vi "SaveDataToDiskAsGlimpse.vi"(0 "Read or Write Path":path, 1 "Array (U8)":u8[][](array[numeric]), 2 "T = AddNewData\nF = if exist, OverWrite or CreateNew":bool=TRUE, 3 "Data type":enum16{"U8", "I16"}(ring), 4 "Array (I16)":i16[][](array[numeric])) -> (8 "error out":errorcluster)   [LabVIEW 2014]
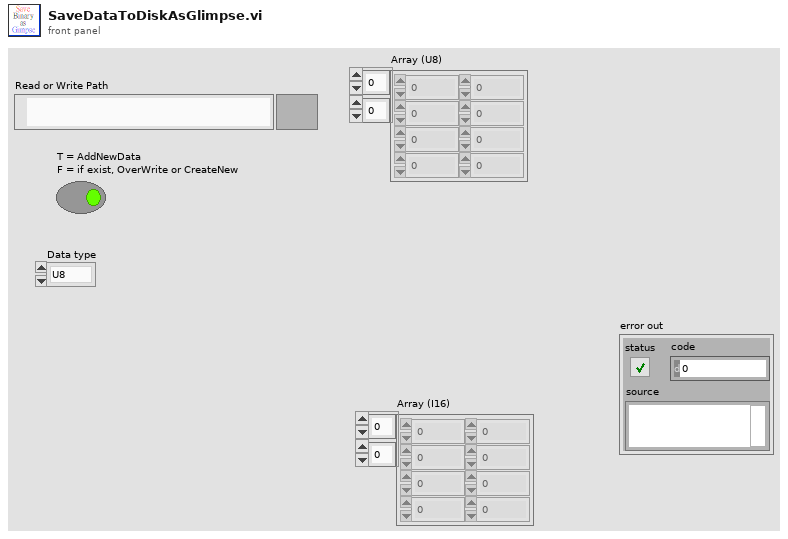
[diagram p1: front panel]
types:
  T1 = enum16{"open", "replace", "create", "open or create", "replace or create", "replace or create with confirmation"}
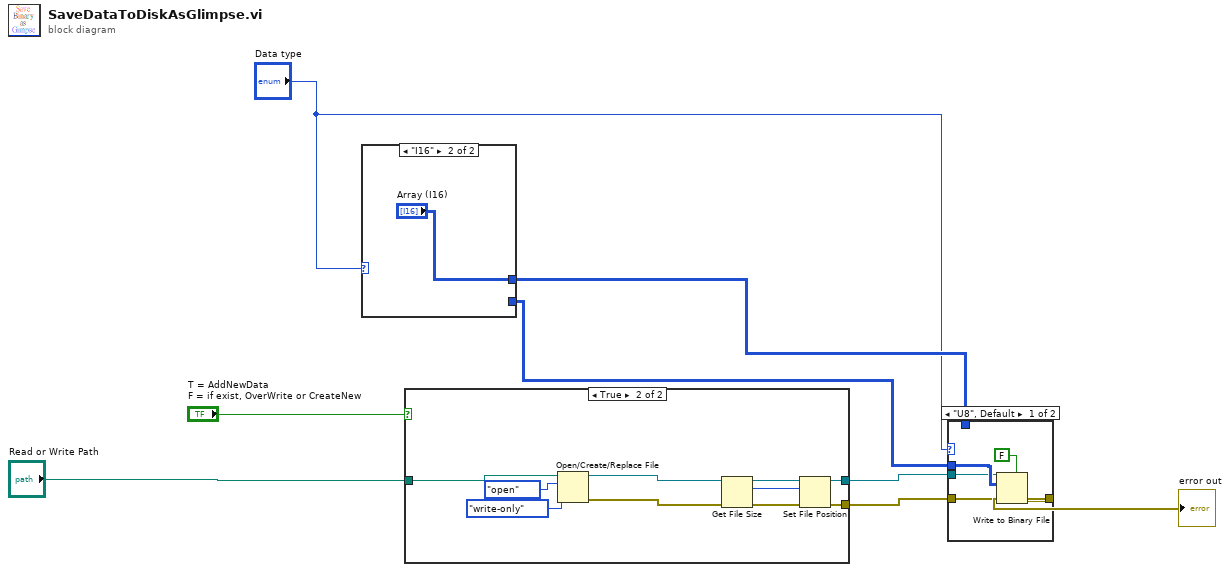
[diagram p0: block diagram]
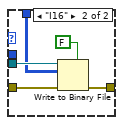
[diagram p2: hidden frame]
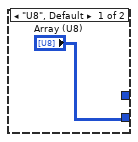
[diagram p3: hidden frame]
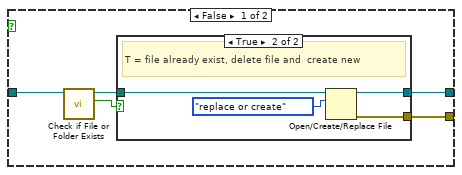
[diagram p4: hidden frame]
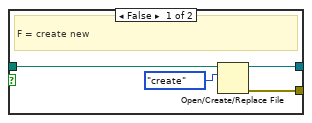
[diagram p5: hidden frame]
diagram:
  n1 = case shown="\"I16\"" "Data type" {
    tunnel: [_ "Array (I16)"] -> w3
    tunnel: ["Array (U8)" _] -> w1
    frame "U8", Default {
    }
    frame "I16" {
    }
  }
  n2 = case shown="True" "T = AddNewData\nF = if exist, OverWrite or CreateNew" {
    tunnel: [w12 w32] -> w7
    tunnel: "Read or Write Path" -> [w15 w28]
    tunnel: [w11 w29] -> w5
    frame False {
      n3 = call <vilib>:"Check if File or Folder Exists.vi"("path"=w15) -> ("file or folder exists?"=w14:bool, "dup path"=w13:path)  [unwired: 8 in, 1 out]
      n4 = case shown="True" w14 {
        tunnel: w13 -> [w19 w22]
        tunnel: [w18 w21] -> w12
        tunnel: [w16 w20] -> w11
        frame False {
          # "F = create new"
          n5 = Open/Create/Replace File(file path (use dialog)=w19, operation (0:open)=T1."create") -> (refnum out=w18:refnum<file>, error out=w16:errorcluster)  [unwired: 4 in, 1 out]
        }
        frame True {
          # "T = file already exist, delete file and  create new"
          n6 = Open/Create/Replace File(file path (use dialog)=w22, operation (0:open)=T1."replace or create") -> (refnum out=w21:refnum<file>, error out=w20:errorcluster)  [unwired: 4 in, 1 out]
        }
      }
    }
    frame True {
      n7 = Open/Create/Replace File(file path (use dialog)=w28, operation (0:open)=T1."open", access (0:read/write)=enum16{"read/write", "read-only", "write-only"}."write-only") -> (refnum out=w26:refnum<file>, error out=w25:errorcluster)  [unwired: 3 in, 1 out]
      n8 = Get File Size(file=w26, error in=w25) -> (refnum out=w33:refnum<file>, size (in bytes)=w31:i64, 0:w30:errorcluster)
      n9 = Set File Position(offset (in bytes) (0)=w31, refnum=w33, error in=w30) -> (refnum out=w32:refnum<file>, error out=w29:errorcluster)  [unwired: 1 in]
    }
  }
  n10 = case shown="\"U8\", Default" "Data type" {
    tunnel: w7 -> [w34 w42]
    tunnel: w5 -> [w36 w41]
    tunnel: [w35 w40] -> w4
    tunnel: w3 -> [_ w39]
    tunnel: w1 -> [w37 _]
    frame "U8", Default {
      n11 = Write to Binary File(file (use dialog)=w34, data=w37, error in=w36, 5:FALSE ("prepend array or string size? (T)")) -> (error out=w35:errorcluster)  [unwired: 2 in, 2 out]
    }
    frame "I16" {
      n12 = Write to Binary File(file (use dialog)=w42, data=w39, error in=w41, 5:FALSE ("prepend array or string size? (T)")) -> (error out=w40:errorcluster)  [unwired: 2 in, 2 out]
    }
  }
  "error out" <- w4
